vi "teste1.vi"() -> ()   [LabVIEW 2020]
panel:
  in  "Boolean 2":bool
  in  "Boolean":bool
  out "btn 4":bool
  out "btn 3":bool
  out "btn 2":bool
  out "btn 1":bool
  in  "VELOCIDADE 100%":bool
  in  "VELOCIDADE 80%":bool
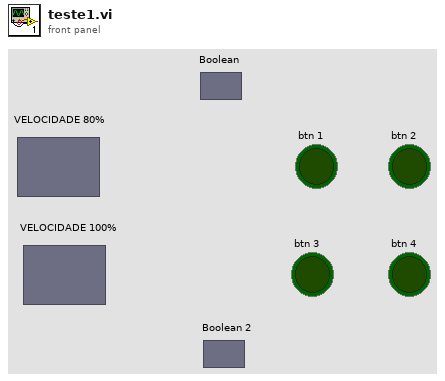
[diagram p1: front panel]
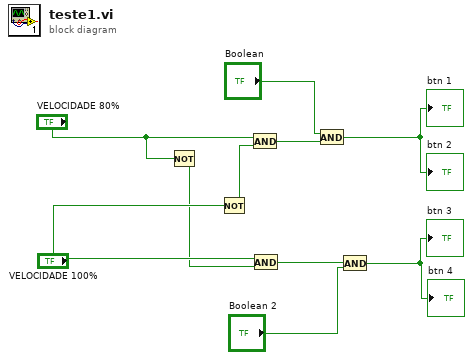
[diagram p0: block diagram]
diagram:
  n1 = Not(x="VELOCIDADE 80%") -> (.not. x?=w7:bool)
  n2 = Not(x="VELOCIDADE 100%") -> (.not. x?=w10:bool)
  n3 = And(x="VELOCIDADE 80%", y=w10) -> (x .and. y?=w3:bool)
  n4 = And(x="VELOCIDADE 100%", y=w7) -> (x .and. y?=w6:bool)
  n5 = And(x="Boolean", y=w3) -> (x .and. y?=→"btn 1" →"btn 2":bool)
  n6 = And(x=w6, y="Boolean 2") -> (x .and. y?=→"btn 3" →"btn 4":bool)
